vi "Single Control Loop.vi"() -> ()   [LabVIEW 2011]
uses:
  <instrlib>/Hokuyo URG Series/Public/Initialize-Standard.vi
  <instrlib>/Hokuyo URG Series/Hokuyo URG Series.lvlib
  <vilib>/robotics/Navigation/shared/WorldMap/OccupancyGridWorldMap/NI_Robotics_OccupancyGridWorldMap.lvclass
panel:
  in  "Step Enable":bool
  out "Error Souce":string
  in  "Resulotion Controller\n1m = 10 units\n30m = 300 units (default)":i32=200
  in  "y Offset":i32
  in  "x Offset":i32
  out "Elapsed Time to Scan for First Time (sec)":dbl
  in  "Step Over":bool
  out "Started Scanning":bool
  out "Occupancy Grid":dbl[][](graph)
  in  "y start":i32
  in  "x start":i32
  out "XY Graph":cluster{dbl[], dbl[]}[](graph)
  in  "ALL STOP":bool
  in  "end point (135°)":dbl=100.0
  in  "start point (-135°)":dbl=-100.0
  in  "VISA resource name":refnum<visa-resource-name>
  # "See the block diagram for modification instructions."
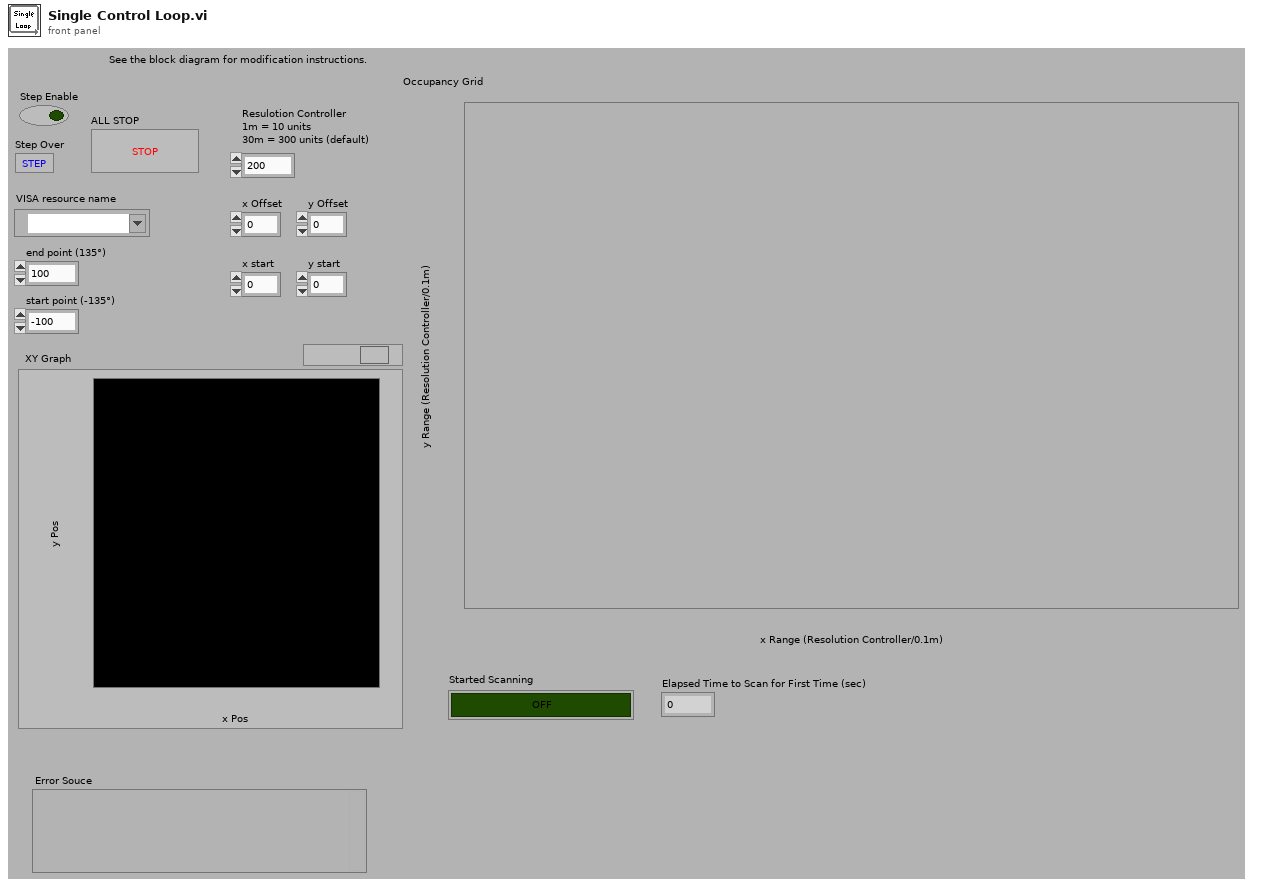
[diagram p1: front panel]
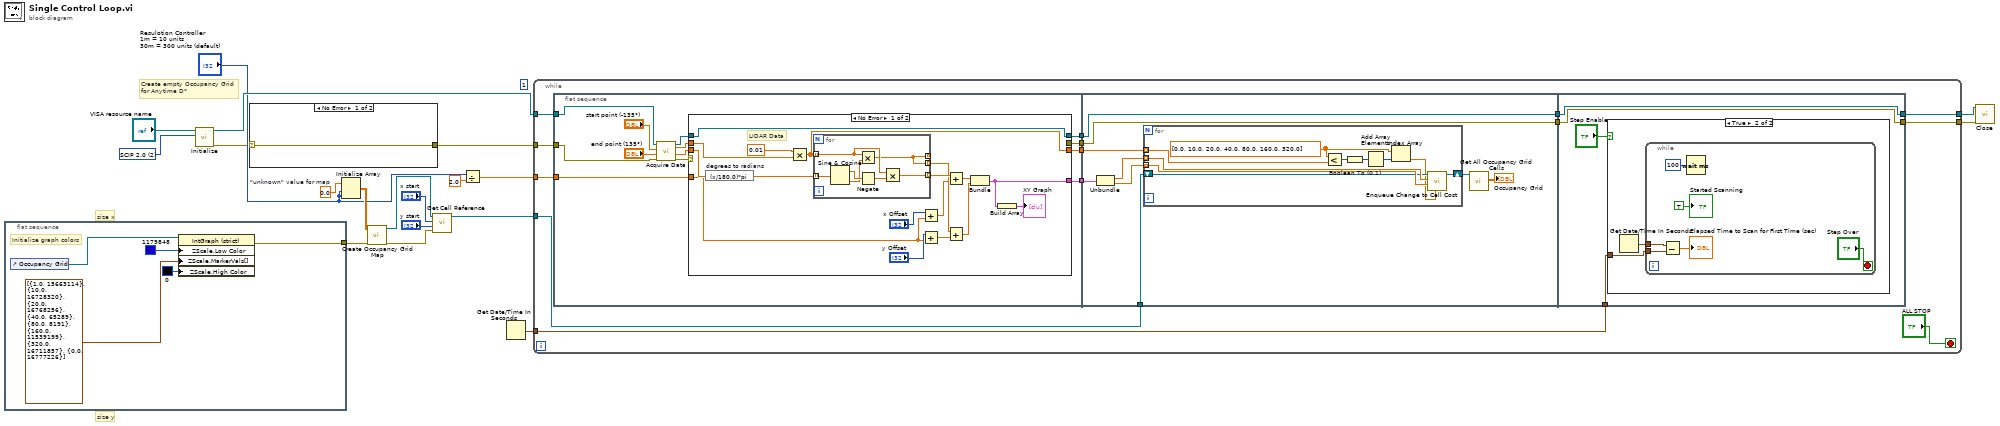
[diagram p0: block diagram]
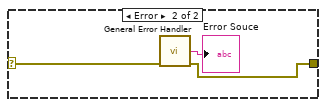
[diagram p4: hidden frame]
diagram:
  (unwired) 1
  w14 = 0.0  # "unknown" value for map
  w15 = u32 2 items=["Convert to Latest", "SCIP 1.1", "SCIP 2.0"] ("Protocol (2: SCIP 2.0)")
  # "size y"
  # "size x"
  # "Create empty Occupancy Grid\nfor Anytime D*"
  n1 = flat-sequence {
    tunnel: [w21] -> w8
    frame #0 {
      # "Initialize graph colors"
      n2 = control-ref of="Occupancy Grid"() -> (w20:refnum<vi>)
      n3 = property on="Property Node" class="IntGraph (strict)"(reference=w20, "ZScale.Low Color"=u32 1179848, "ZScale.MarkerVals[]"=cluster{dbl, u32}[] [{1.0, 15663114}, {10.0, 16728320}, {20.0, 16768256}, {40.0, 65289}, {80.0, 8191}, {160.0, 11539199}, {320.0, 16711857}, {0.0, 16777226}], "ZScale.High Color"=u32 0) -> (error out=w21:errorcluster)  [unwired: 1 in, 1 out]
    }
  }
  n4 = call-poly <instrlib>:"Initialize.vi"("Protocol (2: SCIP 2.0)"=w15, "VISA resource name"="VISA resource name") -> ("error out"=w2:errorcluster, "VISA resource name out"=w18:refnum<visa-resource-name>)  [unwired: 8 in]
  n5 = case shown="No Error" w2 {
    selector: w2 -> [w25 w28]
    tunnel: [w25 w27] -> w1
    frame No Error {
    }
    frame Error {
      n6 = call <vilib>:"General Error Handler.vi"("error in (no error)"=w28) -> ("source out"=→"Error Souce":string, "error out"=w27:errorcluster)  [unwired: 10 in, 3 out]
    }
  }
  n7 = Initialize Array(w14, "Resulotion Controller\n1m = 10 units\n30m = 300 units (default)", "Resulotion Controller\n1m = 10 units\n30m = 300 units (default)") -> (w13:dbl[][])
  n8 = call <vilib>:"Create Occupancy Grid Map.vi"("error in (no error)"=w8, "occupancy grid"=w13) -> ("error out"=w12:errorcluster, "map reference out"=w9:refnum<data-value>)  [unwired: 8 in]
  n9 = call <vilib>:"Get Cell Reference.vi"("error in (no error)"=w12, "y"="y start", "x"="x start", "map reference in"=w9) -> ("map reference out"=w7:refnum<data-value>)  [unwired: 4 in, 3 out]
  n10 = Divide(x="Resulotion Controller\n1m = 10 units\n30m = 300 units (default)", y=2.0) -> (x/y=w4:dbl)
  n11 = Get Date/Time In Seconds() -> (seconds since 1Jan1904=w3:timestamp)
  n12 = while {
    tunnel: w18 -> [w42]
    tunnel: [w37] -> w17
    tunnel: [w41] -> w16
    tunnel: w1 -> [w40]
    tunnel: w7 -> [w36]
    tunnel: w4 -> [w30]
    tunnel: w3 -> [w31]
    stop <- "ALL STOP" stop-if-true
    n13 = flat-sequence {
      tunnel: w42 -> [w49]
      tunnel: w40 -> [w46]
      tunnel: [w48] -> w39
      tunnel: [w47] -> w38
      tunnel: [w45] -> w33
      tunnel: [w44] -> w32
      tunnel: w30 -> [w43]
      tunnel: w39 -> [w90]
      tunnel: w38 -> [w89]
      tunnel: w36 -> [w84]
      tunnel: [w90] -> w35
      tunnel: [w89] -> w34
      tunnel: w33 -> [w82]
      tunnel: w32 -> [w83]
      tunnel: [w103] -> w41
      tunnel: [w104] -> w37
      tunnel: w35 -> [w104]
      tunnel: w34 -> [w103]
      tunnel: w31 -> [w102]
      frame #0 {
        n14 = call <instrlib>:"Acquire Data.vi"("error in (no error)"=w46, "End Point (120°)"="end point (135°)", "Start Point (-120°)"="start point (-135°)", "VISA resource name"=w49) -> ("error out"=w50:errorcluster, "Direction"=w54:dbl[], "Magnitude"=w55:dbl[], "VISA resource name out"=w51:refnum<visa-resource-name>)  [unwired: 4 in]
        n15 = case shown="No Error" w50 {
          selector: w50 -> [_ w80]
          tunnel: w55 -> [w68 _]
          tunnel: w54 -> [w71 _]
          tunnel: w51 -> [w72 w81]
          tunnel: [w72 w81] -> w48
          tunnel: [_ w80] -> w47
          tunnel: [w66 _] -> w45
          tunnel: [w65 _] -> w44
          tunnel: w43 -> [w56 _]
          frame No Error {
            # "LIDAR Data"
            n16 = expression code="(x/180.0)*pi" "degrees to radians"(w71) -> (w70:dbl[])
            n17 = Multiply(x=0.01, y=w68) -> (x*y=w65:dbl[])
            n18 = for {
              tunnel: w65 -> [w74] mode=indexing
              tunnel: w70 -> [w75] mode=indexing
              tunnel: [w77] -> w64 mode=indexing
              tunnel: [w73] -> _ mode=indexing
              tunnel: [w73] -> w62 mode=indexing
              n19 = Sine & Cosine(0:w75) -> (1:w79:dbl, 2:w78:dbl)
              n20 = Multiply(x=w74, y=w78) -> (x*y=w73:dbl)
              n21 = Negate(x=w79) -> (-x=w76:dbl)
              n22 = Multiply(x=w74, y=w76) -> (x*y=w77:dbl)
            }
            n23 = Add(x="x Offset", y=w56) -> (x+y=w60:dbl)
            n24 = Add(x="y Offset", y=w56) -> (x+y=w59:dbl)
            n25 = Add(x=w64, y=w60) -> (x+y=w63:dbl[])
            n26 = Add(x=w62, y=w59) -> (x+y=w61:dbl[])
            n27 = Bundle(w63, w61) -> (w66:cluster{dbl[], dbl[]})  [unwired: 1 out]
            n28 = Build Array(w66) -> (→"XY Graph":cluster{dbl[], dbl[]}[])
          }
          frame Error {
          }
        }
      }
      frame #1 {
        n29 = Unbundle(w82) -> (w85:dbl[], w86:dbl[])
        n30 = for {
          tunnel: w85 -> [w99] mode=indexing
          tunnel: w86 -> [w100] mode=indexing
          shift-right: [w97] -> w87
          shift-left: w84 -> [w98]
          tunnel: w83 -> [w92] mode=indexing
          w93 = dbl[] [0.0, 10.0, 20.0, 40.0, 80.0, 160.0, 320.0]
          n31 = Less?(x=w93, y=w92) -> (x < y?=w91:bool[])
          n32 = Boolean To (0,1)(Boolean=w91) -> (0, 1=w96:i16[])
          n33 = Add Array Elements(numeric array=w96) -> (sum=w95:i16)
          n34 = Index Array(array=w93, index=w95) -> (element=w94:dbl)
          n35 = call <vilib>:"Enqueue Change to Cell Cost.vi"("cost"=w94, "y"=w100, "x"=w99, "map reference in"=w98) -> ("map reference out"=w97:refnum<data-value>)  [unwired: 6 in, 1 out]
        }
        n36 = call <vilib>:"Get All Occupancy Grid Cells.vi"("map reference in"=w87) -> ("occupancy grid"=→"Occupancy Grid":dbl[][])  [unwired: 8 in, 2 out]
      }
      frame #2 {
        n37 = case shown="True" "Step Enable" {
          tunnel: w102 -> [_ w106]
          frame False {
          }
          frame True {
            n38 = Get Date/Time In Seconds() -> (seconds since 1Jan1904=w105:timestamp)
            n39 = while {
              tunnel: w106 -> [w109]
              tunnel: w105 -> [w107]
              stop <- "Step Over" stop-if-true
              n40 = Subtract(x=w107, y=w109) -> (x-y=→"Elapsed Time to Scan for First Time (sec)":dbl)
              n41 = Wait (ms)(milliseconds to wait=u32 100) -> ()  [unwired: 1 out]
              "Started Scanning" <- TRUE ("Boolean")
            }
          }
        }
      }
    }
  }
  n42 = call <instrlib>:"Close.vi"("error in (no error)"=w16, "VISA resource name"=w17) -> ()  [unwired: 9 in, 1 out]
